vi "AO Interupt JSON to Generation Data.vi"(4 "Variant":variant, 6 "File Refnum":refnum<file>, 7 "Data Generation Type":T1, 8 "error in":errorcluster, 9 "1D Waveform Array":waveform(dbl)[](array[waveform]), 10 "1D DBL Array":dbl[](array[numeric]), 11 "Channel Names":string[](array[string])) -> (0 "error out":errorcluster, 2 "1D Waveform Array":waveform(dbl)[](array[waveform]), 3 "1D DBL Array":dbl[](array[numeric]), 5 "Data Generation Type":T1)   [LabVIEW 2024]
doc: "All Rights Reserved © 2017 SyncSols"
uses:
  Controls/AO 1D DBL ArrayCluster.ctl
  Controls/AO Data Gen Type.ctl
  Controls/AO DBL Data Cluster.ctl
  Controls/AO 1D DBL Interface Data Cluster.ctl
  <vilib>/measure/NI_MABase.lvlib
  Controls/AO Sampling Info Cluster.ctl
  Controls/AO 1D Waveform Config Cluster.ctl
  Controls/AO Data Type Identifying Cluster.ctl
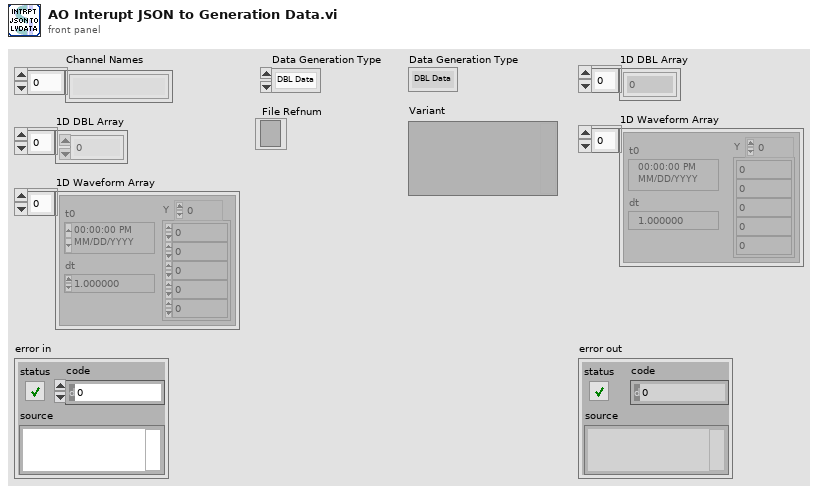
[diagram p1: front panel]
types:
  T1 = typedef "AO Data Gen Type.ctl" = enum16{"DBL Data", "Waveform Data"}
  T2 = typedef "AO Data Type Identifying Cluster.ctl" = cluster{"DBL":T3, "Wave form":T6[], "Data Generation Type":T1}
  T3 = typedef "AO 1D DBL ArrayCluster.ctl" = cluster{"Interface":string, "Interface Data":T4}
  T4 = typedef "AO 1D DBL Interface Data Cluster.ctl" = cluster{"Command":string, "SubCmd":string, "Data":T5[]}
  T5 = typedef "AO DBL Data Cluster.ctl" = cluster{"Channel":string, "Data":dbl}
  T6 = typedef "AO 1D Waveform Config Cluster.ctl" = cluster{"Channel":string, "Pattern":string, "Amplitude":dbl, "frequency":dbl, "Phase":i32, "sampling info":T7}
  T7 = typedef "AO Sampling Info Cluster.ctl" = cluster{"Fs":dbl, "#s":dbl}
  T8 = enum16{"Sine Wave", "Triangle Wave", "Square Wave", "Sawtooth Wave"}
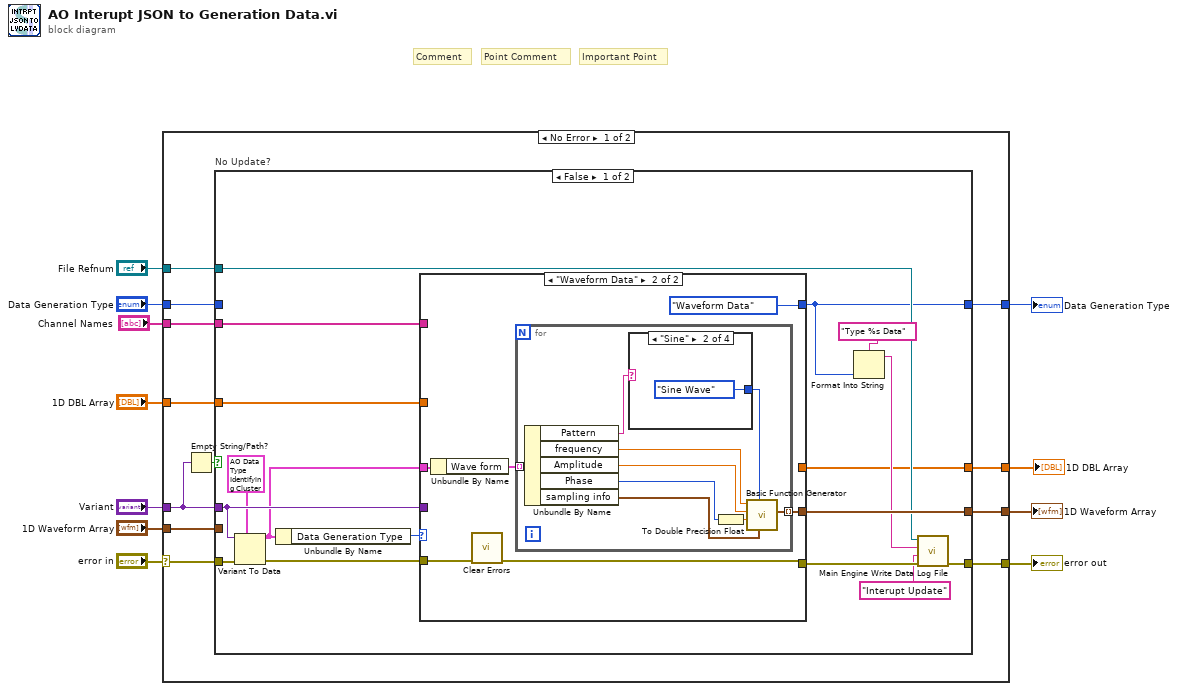
[diagram p0: block diagram]
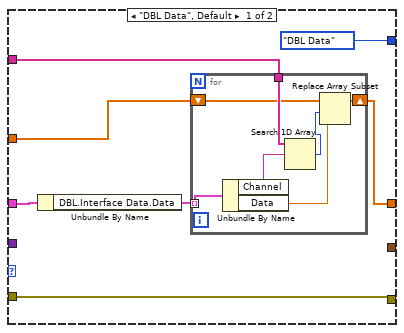
[diagram p2: hidden frame]
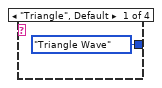
[diagram p3: hidden frame]
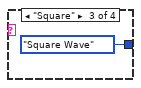
[diagram p4: hidden frame]
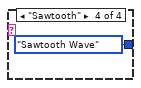
[diagram p5: hidden frame]
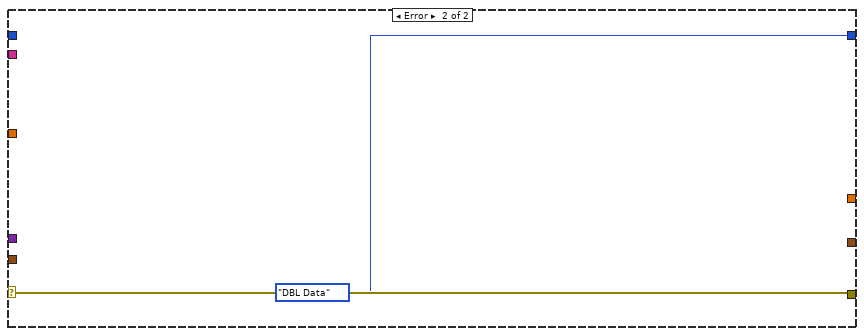
[diagram p7: hidden frame]
diagram:
  # "Important Point"
  # "Point Comment"
  # "Comment"
  n1 = case shown="No Error" "error in" {
    selector: "error in" -> [w23 w79]
    tunnel: [w22 w79] -> w11
    tunnel: "Variant" -> [w18 _]
    tunnel: [w21 AO_Data_Gen_Type."DBL Data" ("Data Generation Type")] -> w9
    tunnel: [w20 _] -> w8
    tunnel: [w19 _] -> w7
    tunnel: "Data Generation Type" -> [w16 _]
    tunnel: "1D DBL Array" -> [w15 _]
    tunnel: "1D Waveform Array" -> [w14 _]
    tunnel: "File Refnum" -> [w13 _]
    tunnel: "Channel Names" -> [w12 _]
    frame No Error {
      n2 = Empty String/Path?(string/path=w18) -> (empty?=w17:bool)
      n3 = case "No Update?" shown="False" w17 {
        tunnel: w23 -> [w31 w77]
        tunnel: [w38 w77] -> w22
        tunnel: [w35 w76] -> w21
        tunnel: [w27 w75] -> w20
        tunnel: w18 -> [w30 _]
        tunnel: [w40 w74] -> w19
        tunnel: w16 -> [_ w76]
        tunnel: w15 -> [w24 w75]
        tunnel: w14 -> [_ w74]
        tunnel: w13 -> [w37 _]
        tunnel: w12 -> [w25 _]
        frame False {
          n4 = Variant To Data(error in=w31, type=T2 {"DBL"={"Interface"="AIO", "Interface Data"={"Command"="Update", "SubCmd"="AO", "Data"=[]}}, "Wave form"=[], "Data Generation Type"=enum."Waveform Data"}, Variant=w30) -> (data=w28:T2, error out=w32:errorcluster)
          n5 = Unbundle By Name(w28) -> ("Data Generation Type"=w26:T1)
          n6 = case shown="\"Waveform Data\"" w26 {
            tunnel: [w47 w57] -> w39
            tunnel: [AO_Data_Gen_Type."DBL Data" ("Data Generation Type") AO_Data_Gen_Type."Waveform Data" ("Data Generation Type")] -> w35
            tunnel: [_ w59] -> w40
            tunnel: w30 -> [_ _]
            tunnel: w32 -> [w47 w58]
            tunnel: w28 -> [w45 w56]
            tunnel: [w43 _] -> w27
            tunnel: w25 -> [w42 _]
            tunnel: w24 -> [w41 _]
            frame "DBL Data", Default {
              n7 = Unbundle By Name(w45) -> ("DBL.Interface Data.Data"=w44:T5[])
              n8 = for {
                tunnel: w44 -> [w54] mode=indexing
                tunnel: w42 -> [w53]
                shift-right: [w48] -> w43
                shift-left: w41 -> [w51]
                n9 = Unbundle By Name(w54) -> ("Channel"=w52:string, "Data"=w49:dbl)
                n10 = Search 1D Array(1D array=w53, element=w52) -> (index of element=w50:i32)  [unwired: 1 in]
                n11 = Replace Array Subset(array=w51, new element=w49, index=w50) -> (w48:dbl[])
              }
            }
            frame "Waveform Data" {
              n12 = Unbundle By Name(w56) -> ("Wave form"=w55:T6[])
              n13 = call <vilib>:"Clear Errors.vi"("error in (no error)"=w58) -> ("error out"=w57:errorcluster)  [unwired: 5 in, 1 out]
              n14 = for {
                tunnel: [w68] -> w59 mode=indexing
                tunnel: w55 -> [w67] mode=indexing
                n15 = Unbundle By Name(w67) -> ("Pattern"=w61:string, "frequency"=w66:dbl, "Amplitude"=w65:dbl, "Phase"=w64:i32, "sampling info"=w62:T7)
                n16 = case shown="\"Sine\"" w61 {
                  tunnel: [T8."Triangle Wave" ("signal type") T8."Sine Wave" ("signal type") T8."Square Wave" ("signal type") T8."Sawtooth Wave" ("signal type")] -> w69
                  frame "Triangle", Default {
                  }
                  frame "Sine" {
                  }
                  frame "Square" {
                  }
                  frame "Sawtooth" {
                  }
                }
                n17 = To Double Precision Float(number=w64) -> (double precision float=w63:dbl)
                n18 = call <vilib>:"Basic Function Generator.vi"("sampling info"=w62, "signal type"=w69, "phase"=w63, "amplitude"=w65, "frequency"=w66) -> ("signal out"=w68:waveform(dbl))  [unwired: 4 in, 2 out]
              }
            }
          }
          n19 = Format Into String(format string="Type %s Data", w35) -> (resulting string=w33:string)  [unwired: 2 in, 1 out]
          n20 = call "Main Engine Write Data Log File.vi"("error in"=w39, "State"="Interupt Update", "Input Data"=w33, "File Refnum"=w37) -> ("error out"=w38:errorcluster)  [unwired: 6 in, 1 out]
        }
        frame True {
        }
      }
    }
    frame Error {
    }
  }
  "error out" <- w11
  "Data Generation Type" <- w9
  "1D DBL Array" <- w8
  "1D Waveform Array" <- w7
